vi "ep_Check Efficiency.vi"(8 "error in (no error)":errorcluster, 11 "efficiency [%]":dbl) -> (0 "error out":errorcluster)   [LabVIEW 2014, in "NI_EP_Motor Monitoring.lvlib"]
uses:
  <vilib>/addons/Electrical Power/Motor Monitoring/NI_EP_Motor Monitoring.lvlib
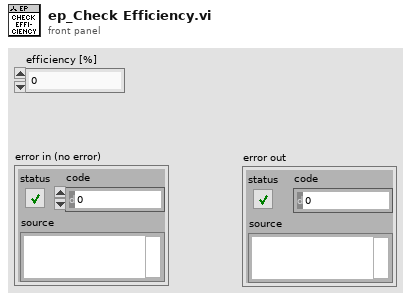
[diagram p1: front panel]
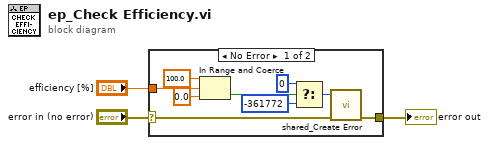
[diagram p0: block diagram]
diagram:
  n1 = case shown="No Error" "error in (no error)" {
    selector: "error in (no error)" -> [w10 w13]
    tunnel: [w9 w13] -> w2
    tunnel: "efficiency [%]" -> [w7 _]
    frame No Error {
      n2 = In Range and Coerce(upper limit=100.0, x=w7, lower limit=0.0) -> (In Range?=w6:bool)  [unwired: 1 out]
      n3 = Select(t=0, s=w6, f=-361772 ("error code (0)")) -> (s? t:f=w8:i32)
      n4 = call <vilib>:"shared_Create Error.vi"("error in (no error)"=w10, "error code (0)"=w8) -> ("error out"=w9:errorcluster)  [unwired: 9 in]
    }
    frame Error {
    }
  }
  "error out" <- w2
